vi "Target Finder.vi"(0 "HSL Range":T7={"Hue"={0.0, 6.122448979591837}, "Saturation"={0.0, 6.122448979591837}, "Luminance"={0.0, 6.122448979591837}} {"Luminance" scale=0.0..255.0; "Saturation" scale=0.0..255.0; "Hue" scale=0.0..255.0}, 1 "Image":T2, 2 "Minimum Area":dbl=1500.0, 4 "Target Selector":dbl, 5 "Mode":T3(ring)=enum."Auto Disabled", 8 "Auton Mode":T1=enum."Second hot target") -> (14 "Thresholded IMage":T2, 16 "Targetssssss":T4)   [LabVIEW 2013]
uses:
  <vilib>/vision/Image Controls.llb/IMAQ Image.ctl
  HSLRange.ctl
  Targetsss.ctl
  Target Type.ctl
  Scores.ctl
  Auton Mode.ctl
panel:
  in  "Score Limits":dbl
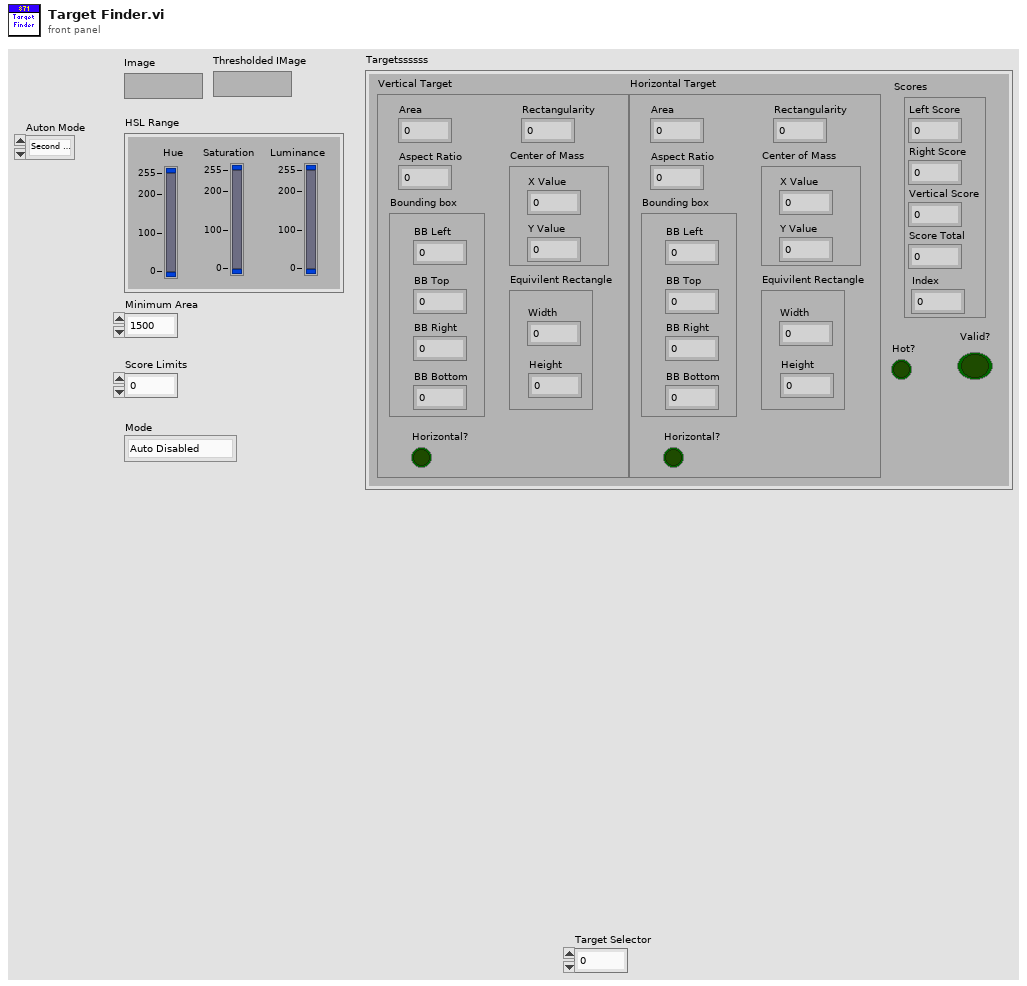
[diagram p1: front panel]
types:
  T1 = typedef "Auton Mode.ctl" = enum16{"Go to closest", "Second hot target", "Go for hot"}
  T2 = typedef "IMAQ Image.ctl" = refnum<image>
  T3 = enum8{"Tele-Op Disabled", "Tele-Op Enabled", "Auto Disabled", "Auto Enabled", "Test Disabled", "Test Enabled", ""}
  T4 = typedef "Targetsss.ctl" = cluster{"Vertical Target":T5, "Horizontal Target":T5, "Valid?":bool, "Scores":T6, "Hot?":bool}
  T5 = typedef "Target Type.ctl" = cluster{"Area":dbl, "Bounding box":cluster{"BB Left":dbl, "BB Top":dbl, "BB Right":dbl, "BB Bottom":dbl}, "Center of Mass":cluster{"X Value":dbl, "Y Value":dbl}, "Equivilent Rectangle":cluster{"Width":dbl, "Height":dbl}, "Aspect Ratio":dbl, "Rectangularity":dbl, "Horizontal?":bool}
  T6 = typedef "Scores.ctl" = cluster{"Score Total":dbl, "Left Score":dbl, "Right Score":dbl, "Vertical Score":dbl, "Index":dbl}
  T7 = typedef "HSLRange.ctl" = cluster{"Hue":cluster{dbl, dbl}, "Saturation":cluster{dbl, dbl}, "Luminance":cluster{dbl, dbl}}
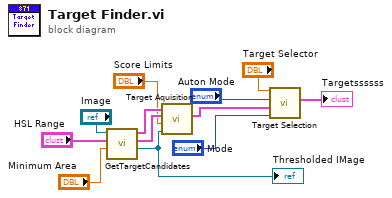
[diagram p0: block diagram]
diagram:
  n1 = call "GetTargetCandidates.vi"("Minimum Area"="Minimum Area", "HSL Range"="HSL Range", "Image"="Image") -> ("Thresholded Image"=w2:T2, "Horizontal Targets"=w7:T5[], "Vertical Targetss"=w8:T5[])  [unwired: 6 in]
  "Thresholded IMage" <- w2
  n2 = call "Target Aquisition.vi"("Image"=w2, "Score Limit"="Score Limits", "Horizontal Targetsssss"=w7, "Vertical Targetsssss"=w8) -> ("Possible Targets"=w6:T4[])  [unwired: 7 in]
  n3 = call "Target Selection.vi"("Mode"="Mode", "Possible Targets"=w6, "Auton Mode"="Auton Mode", "Target Selector"="Target Selector") -> ("Targetssssss"=→"Targetssssss":T4)  [unwired: 6 in, 1 out]
